vi "CH_LM Config Display Mode.vi"(0 "Meter Index":i32, 1 "Display Mode":T3, 2 "Display Submode":T2, 3 "View Mode":T1, 5 "error in (no error)":errorcluster, 7 "Timeout / ms (3000)":i32=3000, 8 "Action (query)":bool, 9 "Lock Timeout / ms (1000)":i32=1000) -> (11 "Lock timed out":bool, 14 "Meter Index":i32, 16 "Display Submode":T2, 17 "View Mode":T1, 19 "error out":errorcluster)   [LabVIEW 2012, in "CH_LM.lvlib"]
doc: "This VI can be used to set/query the display mode."
uses:
  CH_LM.lvlib
  CH_LM Display Submode.ctl
  CH_LM View Mode.ctl
  CH_LM Display Mode.ctl
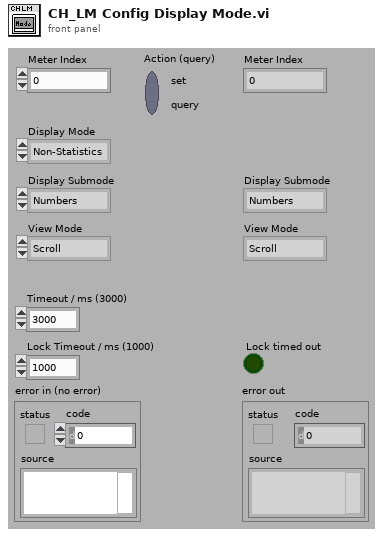
[diagram p1: front panel]
types:
  T1 = typedef "CH_LM.lvlib/CH_LM View Mode.ctl" = enum16{"Scroll", "Fit to Screen", "Strip Chart", "Bar Chart"}
  T2 = typedef "CH_LM.lvlib/CH_LM Display Submode.ctl" = enum16{"Numbers", "Histogram", "Chart"}
  T3 = typedef "CH_LM.lvlib/CH_LM Display Mode.ctl" = enum16{"Non-Statistics", "Statistics", "Position Stability", "Tune", "Trend"}
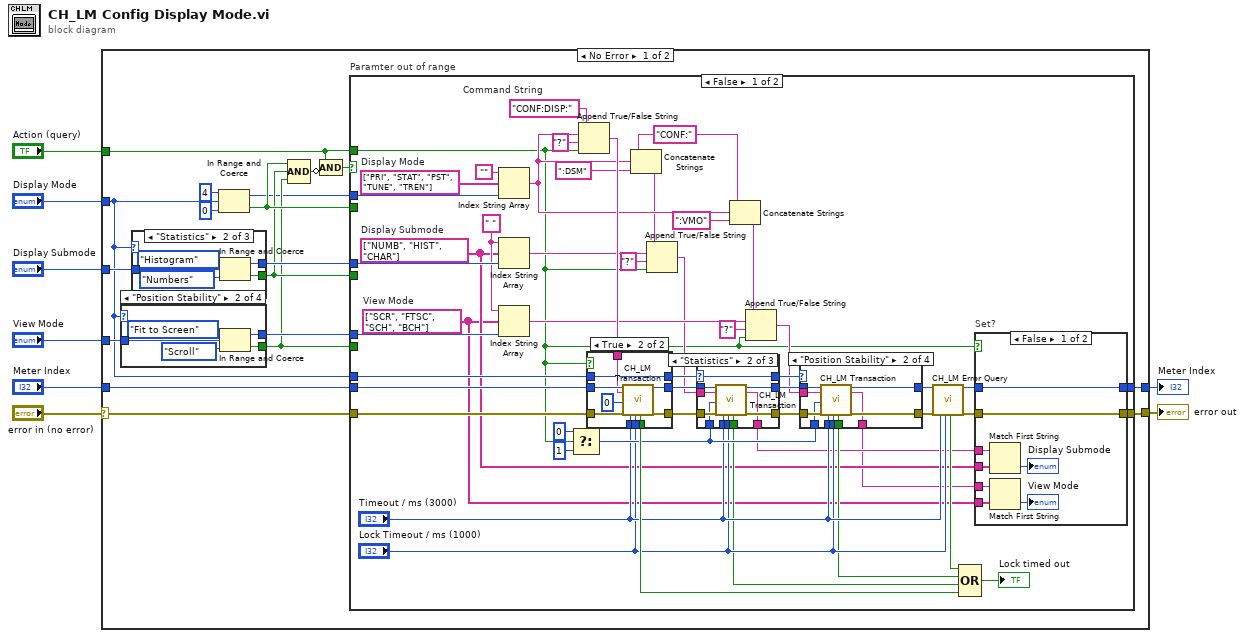
[diagram p0: block diagram]
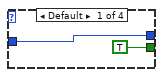
[diagram p2: hidden frame]
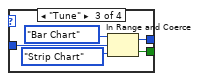
[diagram p3: hidden frame]
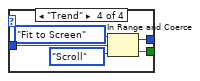
[diagram p4: hidden frame]
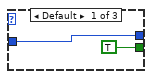
[diagram p5: hidden frame]
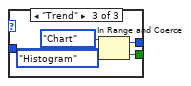
[diagram p6: hidden frame]
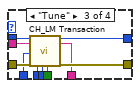
[diagram p9: hidden frame]
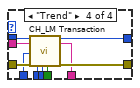
[diagram p10: hidden frame]
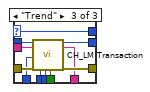
[diagram p12: hidden frame]
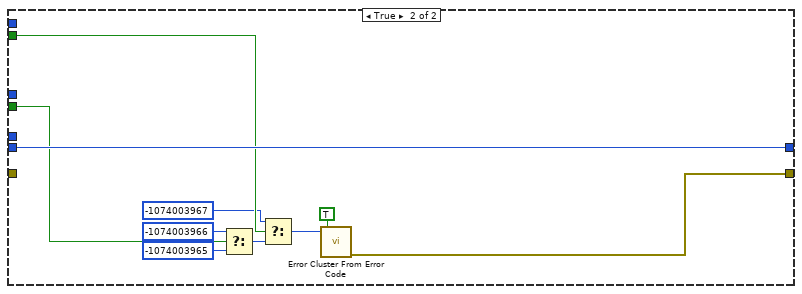
[diagram p14: hidden frame]
diagram:
  n1 = case shown="No Error" "error in (no error)" {
    selector: "error in (no error)" -> [w26 w198]
    tunnel: [w24 w198] -> w8
    tunnel: "Meter Index" -> [w25 w197]
    tunnel: [w23 w197] -> w5
    tunnel: "Action (query)" -> [w22 _]
    tunnel: "Display Mode" -> [w9 _]
    tunnel: "Display Submode" -> [w15 _]
    tunnel: "View Mode" -> [w14 _]
    frame No Error {
      n2 = case shown="\"Position Stability\"" w9 {
        tunnel: [w28 w33 w38 w43] -> w16
        tunnel: w14 -> [w28 w31 w36 w41]
        tunnel: [TRUE w32 w37 w42] -> w11
        frame Default {
        }
        frame "Position Stability" {
          n3 = In Range and Coerce(upper limit=CH_LM_View_Mode."Fit to Screen" ("View Mode"), x=w31, lower limit=CH_LM_View_Mode."Scroll" ("View Mode")) -> (coerced(x)=w33:T1, In Range?=w32:bool)
        }
        frame "Tune" {
          n4 = In Range and Coerce(upper limit=CH_LM_View_Mode."Bar Chart" ("View Mode"), x=w36, lower limit=CH_LM_View_Mode."Strip Chart" ("View Mode")) -> (coerced(x)=w38:T1, In Range?=w37:bool)
        }
        frame "Trend" {
          n5 = In Range and Coerce(upper limit=CH_LM_View_Mode."Fit to Screen" ("View Mode"), x=w41, lower limit=CH_LM_View_Mode."Scroll" ("View Mode")) -> (coerced(x)=w43:T1, In Range?=w42:bool)
        }
      }
      n6 = case shown="\"Statistics\"" w9 {
        tunnel: [w44 w50 w55] -> w17
        tunnel: w15 -> [w44 w49 w54]
        tunnel: [TRUE w48 w53] -> w12
        frame Default {
        }
        frame "Statistics" {
          n7 = In Range and Coerce(upper limit=CH_LM_Display_Submode."Histogram" ("Display Submode"), x=w49, lower limit=CH_LM_Display_Submode."Numbers" ("Display Submode")) -> (coerced(x)=w50:T2, In Range?=w48:bool)
        }
        frame "Trend" {
          n8 = In Range and Coerce(upper limit=CH_LM_Display_Submode."Chart" ("Display Submode"), x=w54, lower limit=CH_LM_Display_Submode."Histogram" ("Display Submode")) -> (coerced(x)=w55:T2, In Range?=w53:bool)
        }
      }
      n9 = In Range and Coerce(upper limit=4, x=w9, lower limit=0) -> (coerced(x)=w10:i32, In Range?=w13:bool)
      n10 = Compound Arithmetic op=AND(w13, w12, w11) -> (w19:bool)
      n11 = Compound Arithmetic op=AND(w22, invert w19) -> (w21:bool)
      n12 = case "Paramter out of range" shown="False" w21 {
        tunnel: w26 -> [w106 _]
        tunnel: w25 -> [w105 w195]
        tunnel: [w95 w194] -> w24
        tunnel: [w93 w195] -> w23
        tunnel: w22 -> [w57 _]
        tunnel: w10 -> [w78 _]
        tunnel: w17 -> [w91 _]
        tunnel: w16 -> [w90 _]
        tunnel: w13 -> [_ _]
        tunnel: w12 -> [_ w189]
        tunnel: w11 -> [_ w193]
        tunnel: w9 -> [w76 _]
        frame False {
          w58 = string[] ["SCR", "FTSC", "SCH", "BCH"]  # View Mode
          w60 = string[] ["NUMB", "HIST", "CHAR"]  # Display Submode
          w92 = string[] ["PRI", "STAT", "PST", "TUNE", "TREN"]  # Display Mode
          w68 = " " ("string (\"\")")
          w73 = "CONF:" ("Command String")
          w101 = "CONF:DISP:"  # Command String
          n13 = Index String Array(1:w78, 2:w92, 3:"") -> (0:w72:string)
          n14 = Index String Array(1:w91, 2:w60, 3:w68) -> (0:w67:string)
          n15 = Index String Array(1:w90, 2:w58, 3:w68) -> (0:w64:string)
          n16 = Select(t=0, s=w57, f=1) -> (s? t:f=w86:i32)
          n17 = Append True/False String(1:w57, 2:"?" ("false string"), 3:w72, 4:w101) -> (0:w99:string)
          n18 = case shown="True" w57 {
            tunnel: w106 -> [w108 w119]
            tunnel: w105 -> [w109 w118]
            tunnel: [_ w117] -> w103
            tunnel: w99 -> [_ w116]
            tunnel: [w108 w115] -> w89
            tunnel: [w109 w113] -> w85
            tunnel: "Timeout / ms (3000)" -> [_ w112]
            tunnel: "Lock Timeout / ms (1000)" -> [_ w111]
            tunnel: w76 -> [w107 w110]
            tunnel: [w107 w110] -> w75
            frame False {
            }
            frame True {
              n19 = call "CH_LM Transaction.vi"("Meter Index"=w118, "Command String"=w116, "NofStrings (-1:all)"=0, "error in (no error)"=w119, "Timeout / ms (3000)"=w112, "Lock Timeout / ms (1000)"=w111) -> ("Lock timed out"=w117:bool, "Meter Index"=w113:i32, "error out"=w115:errorcluster)  [unwired: 11 out]
            }
          }
          n20 = Concatenate Strings(w73, w72, ":DSM" ("Command String")) -> (w69:string)
          n21 = Append True/False String(1:w57, 2:"?" ("false string"), 3:w67, 4:w69) -> (0:w63:string)
          n22 = case shown="\"Statistics\"" w75 {
            selector: w75 -> [w154 w157 w168]
            tunnel: w89 -> [w152 w165 w176]
            tunnel: [w152 w164 w175] -> w88
            tunnel: w86 -> [_ w163 w174]
            tunnel: w85 -> [w153 w162 w173]
            tunnel: [w153 w161 w172] -> w84
            tunnel: "Timeout / ms (3000)" -> [_ w160 w171]
            tunnel: "Lock Timeout / ms (1000)" -> [_ w159 w170]
            tunnel: [_ w158 w169] -> w79
            tunnel: [w154 w157 w168] -> w77
            tunnel: w63 -> [_ w155 w167]
            tunnel: [_ w156 w166] -> w61
            frame Default {
            }
            frame "Statistics" {
              n23 = call "CH_LM Transaction.vi"("Meter Index"=w162, "Command String"=w155, "NofStrings (-1:all)"=w163, "error in (no error)"=w165, "Timeout / ms (3000)"=w160, "Lock Timeout / ms (1000)"=w159) -> ("Lock timed out"=w158:bool, "Meter Index"=w161:i32, "Response"=w156:string, "error out"=w164:errorcluster)  [unwired: 10 out]
            }
            frame "Trend" {
              n24 = call "CH_LM Transaction.vi"("Meter Index"=w173, "Command String"=w167, "NofStrings (-1:all)"=w174, "error in (no error)"=w176, "Timeout / ms (3000)"=w171, "Lock Timeout / ms (1000)"=w170) -> ("Lock timed out"=w169:bool, "Meter Index"=w172:i32, "Response"=w166:string, "error out"=w175:errorcluster)  [unwired: 10 out]
            }
          }
          n25 = Concatenate Strings(w73, w72, ":VMO" ("Command String")) -> (w65:string)
          n26 = Append True/False String(1:w57, 2:"?" ("false string"), 3:w64, 4:w65) -> (0:w62:string)
          n27 = case shown="\"Position Stability\"" w77 {
            tunnel: w88 -> [w120 w131 w141 w151]
            tunnel: [w120 w130 w140 w150] -> w87
            tunnel: w86 -> [_ w129 w139 w149]
            tunnel: w84 -> [w121 w128 w138 w148]
            tunnel: [w121 w127 w137 w147] -> w83
            tunnel: "Timeout / ms (3000)" -> [_ w126 w136 w146]
            tunnel: "Lock Timeout / ms (1000)" -> [_ w125 w135 w145]
            tunnel: [_ w124 w134 w144] -> w80
            tunnel: w62 -> [_ w123 w133 w142]
            tunnel: [_ w122 w132 w143] -> w59
            frame Default {
            }
            frame "Position Stability" {
              n28 = call "CH_LM Transaction.vi"("Meter Index"=w128, "Command String"=w123, "NofStrings (-1:all)"=w129, "error in (no error)"=w131, "Timeout / ms (3000)"=w126, "Lock Timeout / ms (1000)"=w125) -> ("Lock timed out"=w124:bool, "Meter Index"=w127:i32, "Response"=w122:string, "error out"=w130:errorcluster)  [unwired: 10 out]
            }
            frame "Tune" {
              n29 = call "CH_LM Transaction.vi"("Meter Index"=w138, "Command String"=w133, "NofStrings (-1:all)"=w139, "error in (no error)"=w141, "Timeout / ms (3000)"=w136, "Lock Timeout / ms (1000)"=w135) -> ("Lock timed out"=w134:bool, "Meter Index"=w137:i32, "Response"=w132:string, "error out"=w140:errorcluster)  [unwired: 10 out]
            }
            frame "Trend" {
              n30 = call "CH_LM Transaction.vi"("Meter Index"=w148, "Command String"=w142, "NofStrings (-1:all)"=w149, "error in (no error)"=w151, "Timeout / ms (3000)"=w146, "Lock Timeout / ms (1000)"=w145) -> ("Lock timed out"=w144:bool, "Meter Index"=w147:i32, "Response"=w143:string, "error out"=w150:errorcluster)  [unwired: 10 out]
            }
          }
          n31 = call "CH_LM Error Query.vi"("Meter Index"=w83, "error in (no error)"=w87, "Timeout / ms (3000)"="Timeout / ms (3000)", "Lock Timeout / ms (1000)"="Lock Timeout / ms (1000)") -> ("Lock timed out"=w104:bool, "Meter Index"=w94:i32, "error out"=w96:errorcluster)  [unwired: 13 out]
          n32 = Compound Arithmetic op=OR(w104, w80, w79, w103) -> (→"Lock timed out":bool)
          n33 = case "Set?" shown="False" w57 {
            tunnel: w96 -> [w183 w185]
            tunnel: [w183 w185] -> w95
            tunnel: w94 -> [w184 w186]
            tunnel: [w184 w186] -> w93
            tunnel: w61 -> [w182 _]
            tunnel: w60 -> [w181 _]
            tunnel: w59 -> [w180 _]
            tunnel: w58 -> [w179 _]
            frame False {
              n34 = Match First String(2:w181, 3:w182) -> (0:→"Display Submode":i32)  [unwired: 1 out]
              n35 = Match First String(2:w179, 3:w180) -> (0:→"View Mode":i32)  [unwired: 1 out]
            }
            frame True {
            }
          }
        }
        frame True {
          n36 = Select(t=-1074003966 ("error code (0)"), s=w193, f=-1074003965 ("error code (0)")) -> (s? t:f=w190:i32)
          n37 = Select(t=-1074003967 ("error code (0)"), s=w189, f=w190) -> (s? t:f=w187:i32)
          n38 = call <vilib>:"Error Cluster From Error Code.vi"("show call chain? (False)"=TRUE, "error code (0)"=w187) -> ("error out"=w194:errorcluster)  [unwired: 1 in, 6 out]
        }
      }
    }
    frame Error {
    }
  }
  "error out" <- w8
  "Meter Index" <- w5
